vi "Digital input.vi"(8 "error in":errorcluster, 11 "DAQmx InPut Setting":T1) -> (0 "error out":errorcluster, 1 "Exit":bool)   [LabVIEW 2015]
uses:
  <vilib>/DAQmx/read.llb/DAQmx Read (Digital 1D Bool 1Chan 1Samp).vi
  <vilib>/DAQmx/create/channels.llb/DAQmx Create Channel (DI-Digital Input).vi
  Galobal variable_TI.vi
  <vilib>/DAQmx/miscellaneous.llb/DAQmx Fill In Error Info.vi
panel:
  out "error out 2":errorcluster
  out "DAQmx InPut_00":string
  out "*(type *) &x":tag
  out "status":bool
  out "Array":bool[](array[boolean])
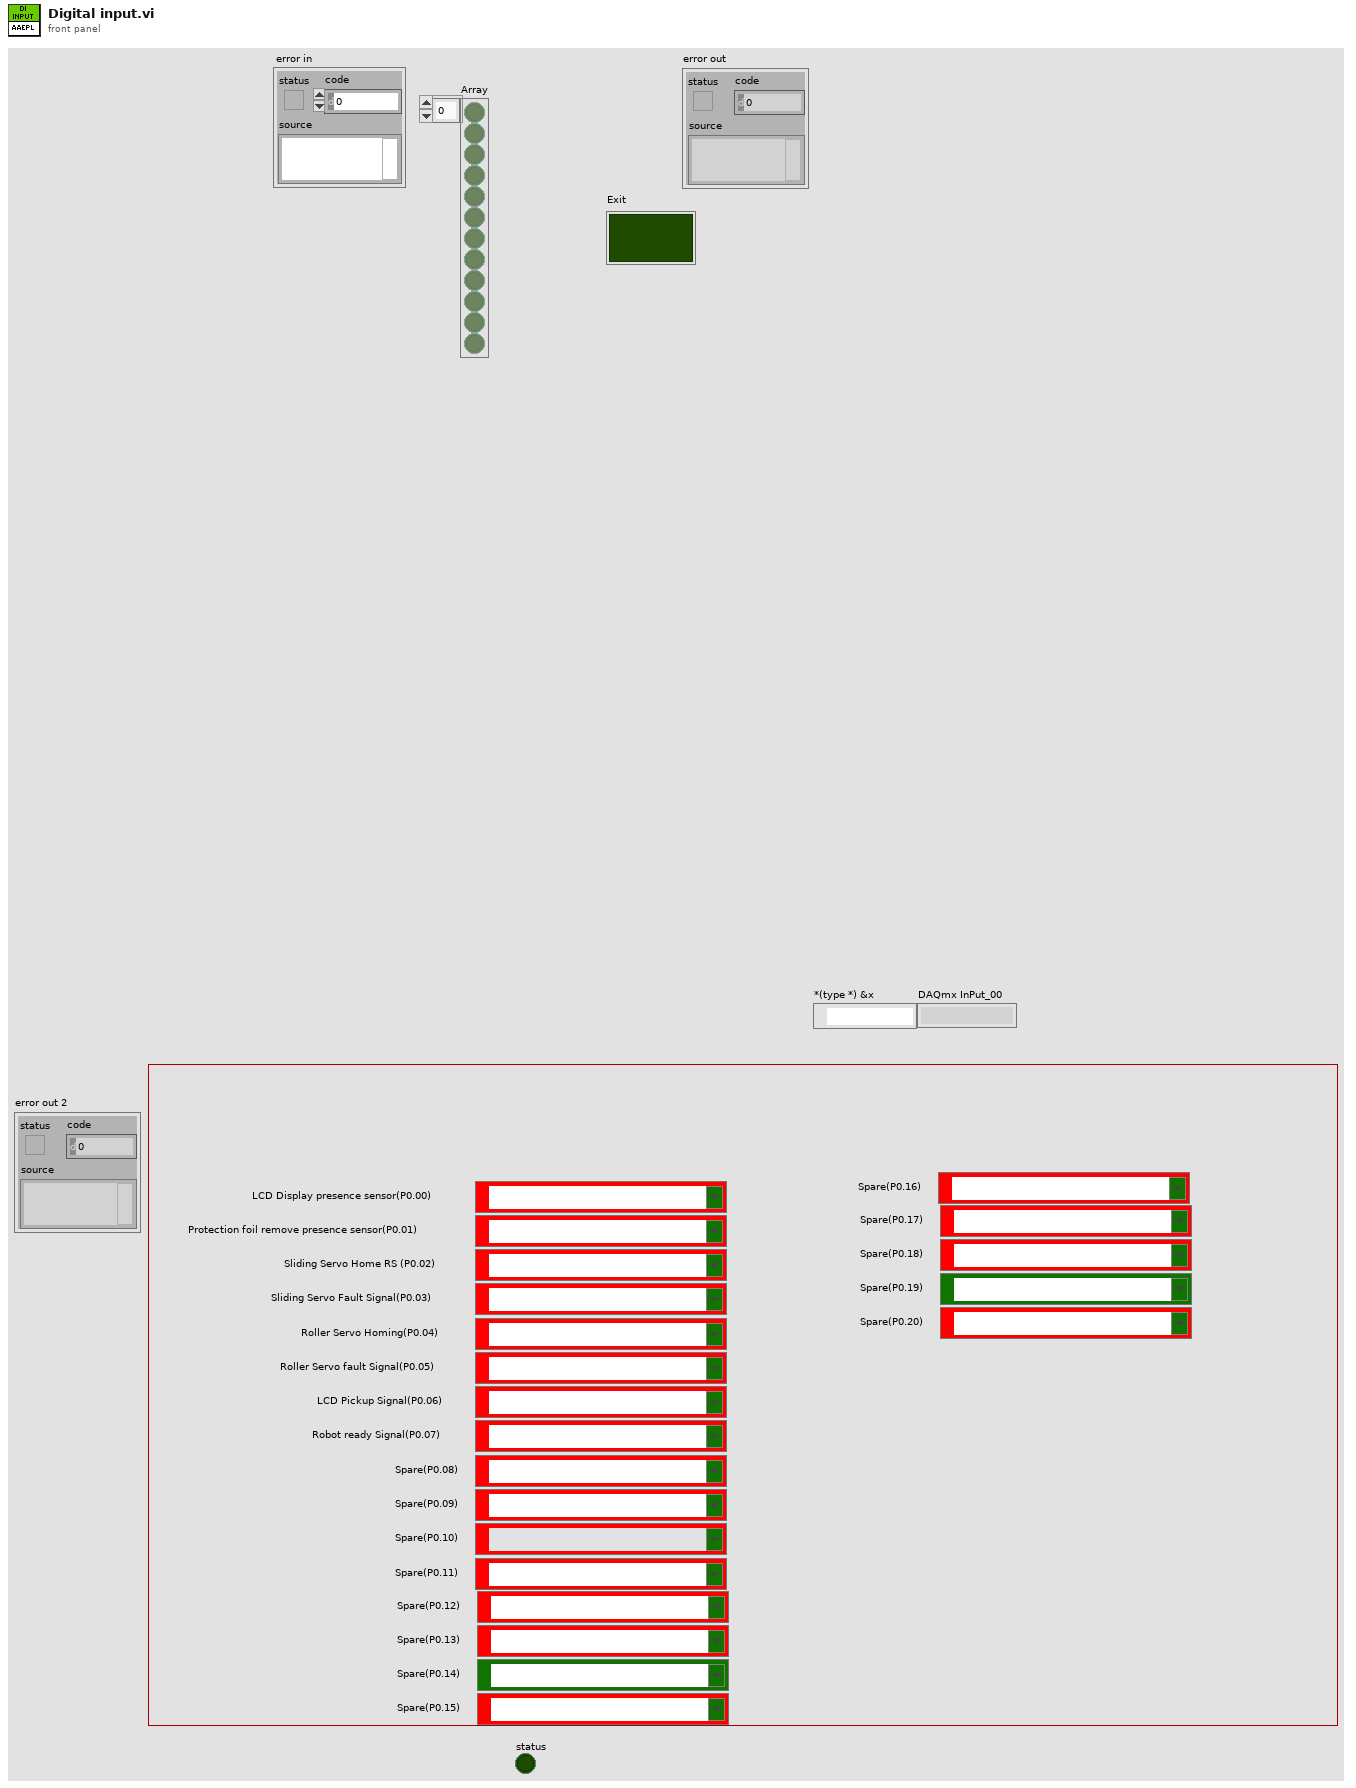
[diagram p1: front panel]
types:
  T1 = cluster{"DAQmx InPut_00":tag, "DAQmx InPut_01":tag, "DAQmx InPut_02":tag, "DAQmx InPut_03":tag, "DAQmx InPut_04":tag, "DAQmx InPut_05":tag, "DAQmx InPut_06":tag, "DAQmx InPut_07":tag, "DAQmx InPut_08":tag, "DAQmx InPut_09":tag, "DAQmx InPut_10":tag, "DAQmx InPut_11":tag, "DAQmx InPut_12":tag, "DAQmx InPut_13":tag, "DAQmx InPut_14":tag, "DAQmx InPut_15":tag, "DAQmx InPut_11 2":tag, "DAQmx InPut_12 2":tag, "DAQmx InPut_13 2":tag, "DAQmx InPut_14 2":tag, "DAQmx InPut_15 2":tag}
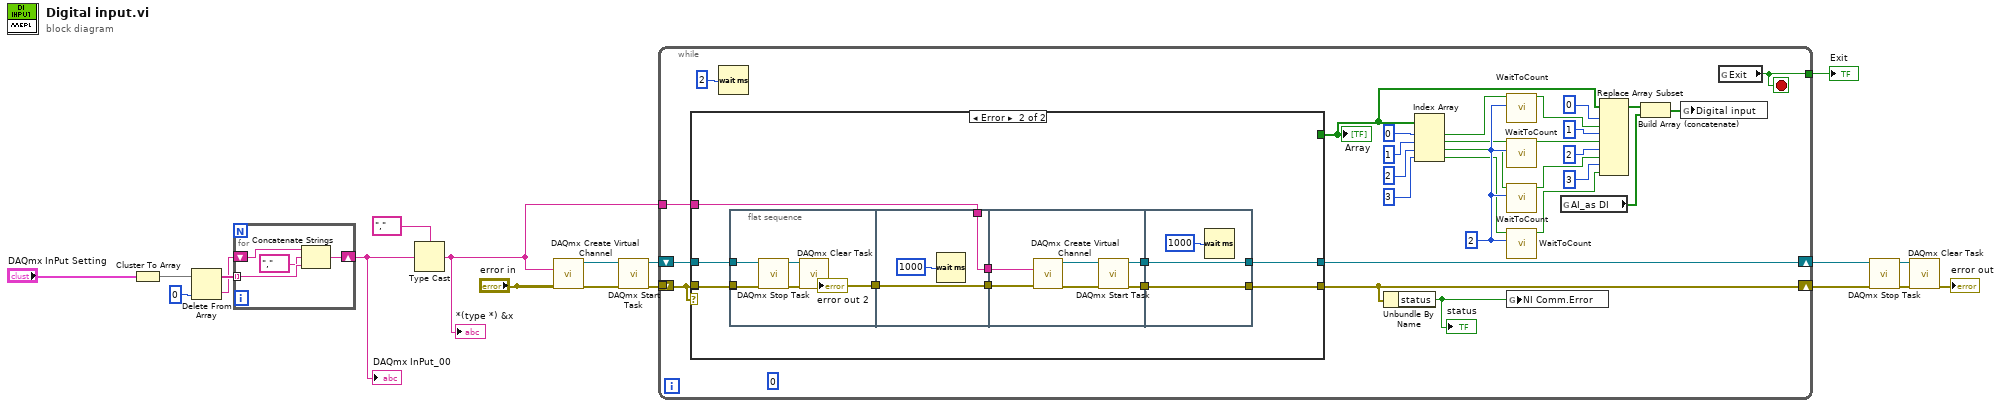
[diagram p0: block diagram]
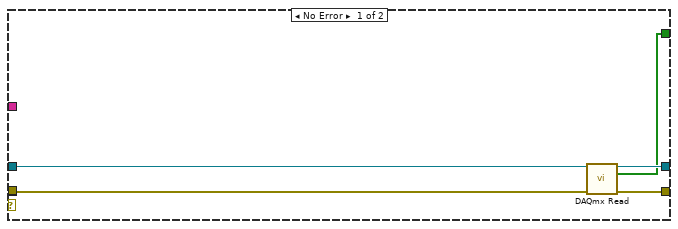
[diagram p2: hidden frame]
diagram:
  n1 = Cluster To Array(cluster="DAQmx InPut Setting") -> (array=w10:tag[])
  n2 = Delete From Array(array=w10, index=0) -> (deleted portion=w7:tag, array with subset deleted=w9:tag[])  [unwired: 1 in]
  n3 = for {
    tunnel: w9 -> [w22] mode=indexing
    shift-right: [w20] -> w5
    shift-left: w7 -> [w23]
    n4 = Concatenate Strings(w23, tag "," ("1."), w22) -> (w20:string)
  }
  "DAQmx InPut_00" <- w5
  n5 = Type Cast(type=tag "," ("1."), x=w5) -> (*(type *) &x=w4:tag)
  "*(type *) &x" <- w4
  n6 = call-poly <vilib>:"DAQmx Create Virtual Channel.vi"("lines"=w4, "error in"="error in") -> ("task out"=w19:refnum<k21>, "error out"=w18:errorcluster)  [unwired: 3 in, 9 out]
  n7 = call <vilib>:"DAQmx Start Task.vi"("task/channels in"=w19, "error in"=w18) -> ("task out"=w16:refnum<k21>, "error out"=w17:errorcluster)  [unwired: 12 out]
  n8 = while {
    shift-right: [w47] -> w13
    shift-left: w17 -> [w53]
    shift-right: [w51] -> w12
    shift-left: w16 -> [w52]
    tunnel: w4 -> [w50]
    tunnel: [w49] -> w11
    tunnel: "error in" -> [w24]
    stop <- w49 stop-if-true
    (unwired) 0 ("Boolean-01 Count")
    w38 = 2 ("Count")
    n9 = case shown="Error" w53 {
      tunnel: w53 -> [w58 w68]
      tunnel: w52 -> [w57 w69]
      tunnel: [w56 w63] -> w47
      tunnel: [w55 w62] -> w51
      tunnel: w50 -> [_ w66]
      tunnel: [w54 _] -> w26
      tunnel: w24 -> [_ w59]
      frame No Error {
        n10 = call-poly <vilib>:"DAQmx Read.vi"("task/channels in"=w57, "error in"=w58) -> ("task out"=w55:refnum<k21>, "data"=w54:bool[], "error out"=w56:errorcluster)  [unwired: 1 in, 10 out]
      }
      frame Error {
        n11 = flat-sequence {
          tunnel: w69 -> [w73]
          tunnel: w68 -> [w72]
          tunnel: [w70] -> w60
          tunnel: w59 -> [w70]
          tunnel: [w77] -> w67
          tunnel: w66 -> [w77]
          tunnel: [w76] -> w61
          tunnel: w60 -> [w76]
          tunnel: w67 -> [w82]
          tunnel: [w81] -> w65
          tunnel: [w80] -> w64
          tunnel: w61 -> [w79]
          tunnel: w65 -> [w87]
          tunnel: w64 -> [w86]
          tunnel: [w87] -> w63
          tunnel: [w86] -> w62
          frame #0 {
            n12 = call <vilib>:"DAQmx Stop Task.vi"("task/channels in"=w73, "error in"=w72) -> ("task out"=w74:refnum<k21>, "error out"=w75:errorcluster)  [unwired: 12 in]
            n13 = call <vilib>:"DAQmx Clear Task.vi"("task in"=w74, "error in"=w75) -> ("error out"=→"error out 2":errorcluster)  [unwired: 13 in]
          }
          frame #1 {
            n14 = Wait (ms)(milliseconds to wait=u32 1000) -> ()  [unwired: 1 out]
          }
          frame #2 {
            n15 = call-poly <vilib>:"DAQmx Create Virtual Channel.vi"("lines"=w82, "error in"=w79) -> ("task out"=w83:refnum<k21>, "error out"=w84:errorcluster)  [unwired: 3 in, 9 out]
            n16 = call <vilib>:"DAQmx Start Task.vi"("task/channels in"=w83, "error in"=w84) -> ("task out"=w80:refnum<k21>, "error out"=w81:errorcluster)  [unwired: 12 out]
          }
          frame #3 {
            n17 = Wait (ms)(milliseconds to wait=u32 1000) -> ()  [unwired: 1 out]
          }
        }
      }
    }
    "Array" <- w26
    n18 = Wait (ms)(milliseconds to wait=u32 2) -> ()  [unwired: 1 out]
    n19 = Unbundle By Name(w47) -> ("status"=w46:bool)
    "status" <- w46
    n20 = Index Array(array=w26, index #1=0 ("index"), index #2=1 ("index"), index #3=2 ("index"), index #4=3 ("index")) -> (element #1=w34:bool, element #2=w35:bool, element #3=w36:bool, element #4=w37:bool)
    n21 = call "WaitToCount.vi"("Count"=w38, "Boolean-01"=w34) -> ("Boolean-01-Indicator"=w39:bool)  [unwired: 8 in, 1 out]
    n22 = call "WaitToCount.vi"("Count"=w38, "Boolean-01"=w35) -> ("Boolean-01-Indicator"=w40:bool)  [unwired: 8 in, 1 out]
    n23 = call "WaitToCount.vi"("Count"=w38, "Boolean-01"=w36) -> ("Boolean-01-Indicator"=w42:bool)  [unwired: 8 in, 1 out]
    n24 = call "WaitToCount.vi"("Count"=w38, "Boolean-01"=w37) -> ("Boolean-01-Indicator"=w43:bool)  [unwired: 8 in, 1 out]
    n25 = global write "Galobal variable_TI.vi" "NI Comm.Error"(w46) -> ()
    n26 = global read "Galobal variable_TI.vi" "AI_as DI"() -> (w48:bool[])
    n27 = Replace Array Subset(array=w26, new element #1=w39, index #1=0 ("index"), new element #2=w40, index #2=1 ("index"), new element #3=w42, index #3=2 ("index"), new element #4=w43, index #4=3 ("index")) -> (w25:bool[])
    n28 = Build Array (concatenate)(w25, w48) -> (w45:bool[])
    n29 = global write "Galobal variable_TI.vi" "Digital input"(w45) -> ()
    n30 = global read "Galobal variable_TI.vi" "Exit"() -> (w49:bool)
  }
  "Exit" <- w11
  n31 = call <vilib>:"DAQmx Stop Task.vi"("task/channels in"=w12, "error in"=w13) -> ("task out"=w14:refnum<k21>, "error out"=w15:errorcluster)  [unwired: 12 in]
  n32 = call <vilib>:"DAQmx Clear Task.vi"("task in"=w14, "error in"=w15) -> ("error out"=→"error out":errorcluster)  [unwired: 13 in]
